vi "niRFUtil FTW Generate Lagrange Interpolation FD Filter.vi"(0 "Half Length":i32=5, 1 "Sampling Rate (Hz)":dbl=1.0 format="%^.3e", 2 "Delay (s)":dbl=5.5 format="%^.3e") -> (14 "Filter":T1 {"y" min=0 max=127 format="%.2f"; "dx" format="%^.2e"; "x0" format="%^.2e"})   [LabVIEW 2015, in "niRFUtil.lvlib"]
uses:
  niRFUtil.lvlib
  Includes/niRFUtil INC Real Waveform.ctl
  Includes/niRFUtil INC Real Array.ctl
  <vilib>/Analysis/NI_AALPro.lvlib
  <vilib>/Analysis/2dsp.llb/Real FFT.vi
panel:
  out "Phase (deg)":cluster{dbl, dbl, dbl[]}(graph)
  out "Mag (dB)":cluster{dbl, dbl, dbl[]}(graph)
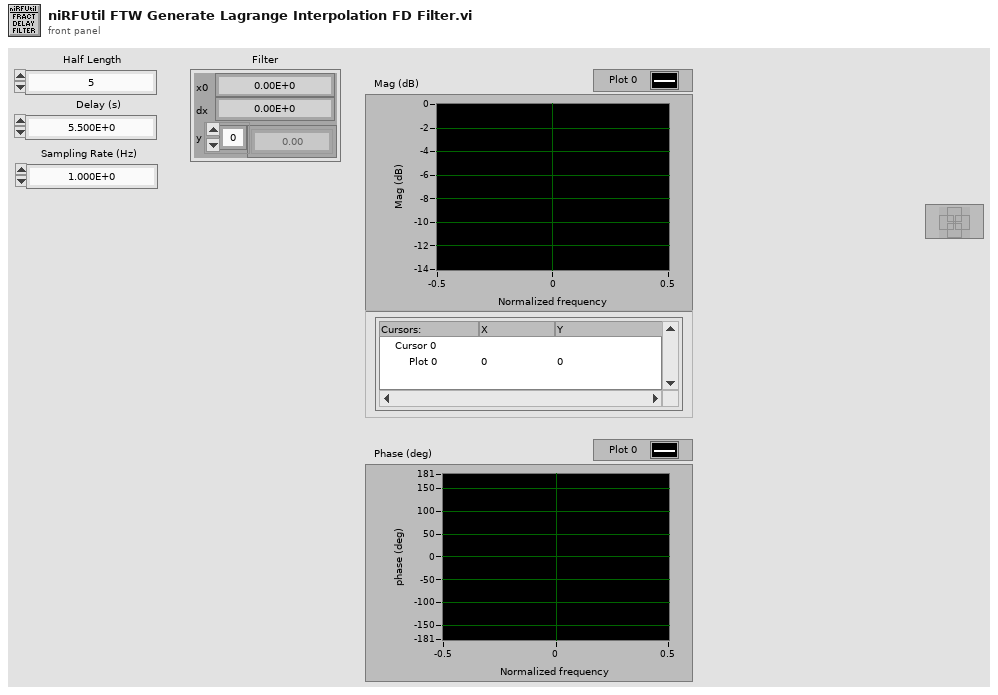
[diagram p1: front panel]
types:
  T1 = typedef "niRFUtil.lvlib/niRFUtil INC Real Waveform.ctl" = cluster{"x0":dbl, "dx":dbl, "y":T2}
  T2 = typedef "niRFUtil.lvlib/niRFUtil INC Real Array.ctl" = sgl[]
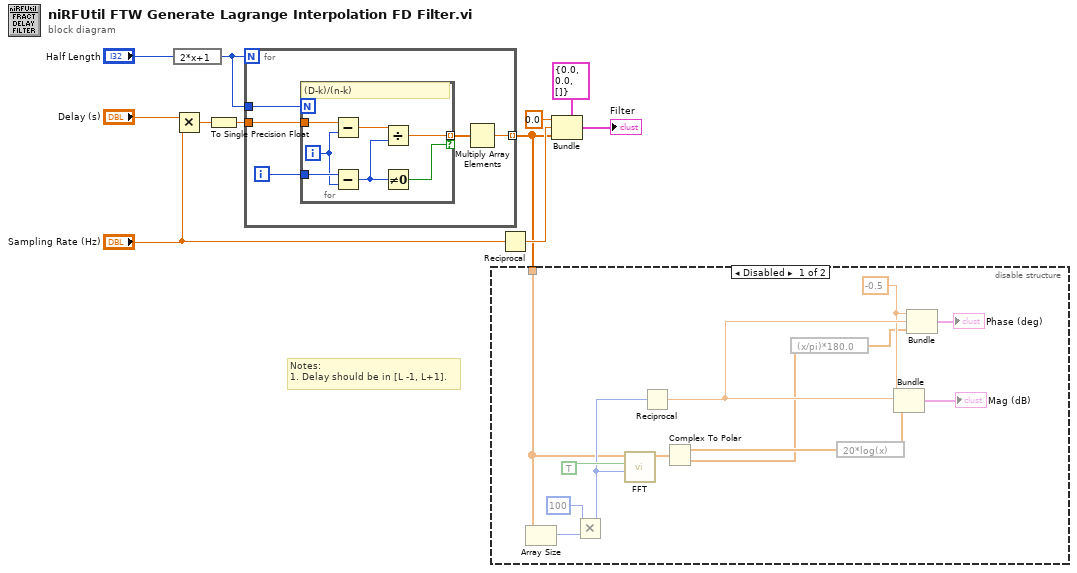
[diagram p0: block diagram]
diagram:
  # "Notes:\n1. Delay should be in [L -1, L+1]."
  n1 = expression code="2*x+1"("Half Length") -> (w11:i32)
  n2 = Multiply(x="Delay (s)", y="Sampling Rate (Hz)") -> (x*y=w8:dbl)
  n3 = To Single Precision Float(number=w8) -> (single precision float=w2:sgl)
  n4 = for {
    N: w11 -> [_]
    tunnel: w2 -> [w16]
    tunnel: w11 -> [w15]
    tunnel: [w12] -> w1 mode=indexing
    i -> [w14]
    n5 = for {
      N: w15 -> [_]
      tunnel: w16 -> [w23]
      tunnel: [w21] -> w13 mode=indexing if=w17
      tunnel: w14 -> [w20]
      i -> [w19]
      # "(D-k)/(n-k)"
      n6 = Subtract(x=w23, y=w19) -> (x-y=w22:sgl)
      n7 = Subtract(x=w20, y=w19) -> (x-y=w18:i32)
      n8 = Divide(x=w22, y=w18) -> (x/y=w21:sgl)
      n9 = Not Equal To 0?(x=w18) -> (x != 0?=w17:bool)
    }
    n10 = Multiply Array Elements(1:w13) -> (0:w12:sgl)
  }
  n11 = disable-structure shown="Disabled" {
    disable-tunnel: w1 -> [w29 _]
    frame Disabled {
      w28 = -0.5
      n12 = Array Size(array=w29) -> (size(s)=w34:i32)
      n13 = Multiply(x=100, y=w34) -> (x*y=w30:i32)
      n14 = call-poly <vilib>:"FFT.vi"("FFT size"=w30, "shift?"=TRUE, "X"=w29) -> ("FFT {X}"=w36:cdb[])  [unwired: 7 in, 1 out]
      n15 = Reciprocal(x=w30) -> (1/x=w31:dbl)
      n16 = Complex To Polar(r * e^(i*theta)=w36) -> (r=w37:dbl[], theta=w25:dbl[])
      n17 = expression code="(x/pi)*180.0" ("radians to degrees")(w25) -> (w24:dbl[])
      n18 = expression code="20*log(x)"(w37) -> (w32:dbl[])
      n19 = Bundle(w28, w31, w32) -> (→"Mag (dB)":cluster{dbl, dbl, dbl[]})  [unwired: 1 in]
      n20 = Bundle(w28, w31, w24) -> (→"Phase (deg)":cluster{dbl, dbl, dbl[]})  [unwired: 1 in]
    }
    frame Enabled {
    }
  }
  n21 = Reciprocal(x="Sampling Rate (Hz)") -> (1/x=w5:dbl)
  n22 = Bundle(cluster=T1 {"x0"=0.0, "dx"=0.0, "y"=[]} ("Filter"), "x0"=0.0, "dx"=w5, "y"=w1) -> (→"Filter":T1)
